vi "destroy.vi"(8 "error in (no error)":errorcluster, 11 "reqwest":refnum<class "reqwest.lvclass">) -> (0 "error out":errorcluster)   [LabVIEW 2020, in "reqwest.lvclass"]
uses:
  reqwest.lvclass
  reqwest.lvclass/reqwest.ctl
  shared-library/reqwest-labview.lvlib
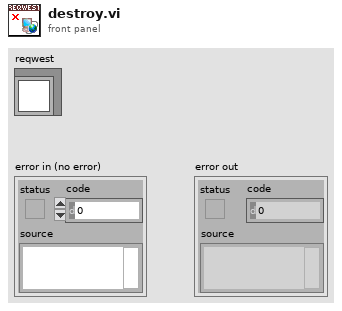
[diagram p1: front panel]
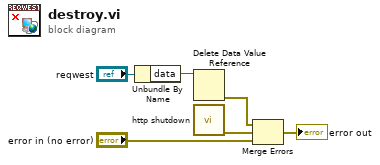
[diagram p0: block diagram]
diagram:
  n1 = Unbundle By Name("reqwest") -> ("data"=w5:refnum<data-value>)
  n2 = Delete Data Value Reference(data value reference=w5) -> (error out=w4:errorcluster)  [unwired: 1 in, 1 out]
  n3 = call "http shutdown.vi"() -> ("error out"=w3:errorcluster)  [unwired: 11 in]
  n4 = Merge Errors(w4, w3, "error in (no error)") -> (→"error out":errorcluster)
